vi "Open Port.vi"(7 "timeout":u32=1000, 8 "error in":errorcluster, 9 "Message Cfg":T1={"EnTermChar"=TRUE, "termChar"=10, "suppEnEnRd"=FALSE, "sendEndEn"=FALSE} {"termChar" format="%.0x"}, 10 "serialCfg":T2={"baud rate (9600)"=9600, "data bits (8)"=8, "stop bits (10: 1 bit)"=10, "parity (0:none)"=enum."None", "flow control (0:none)"=0, "endModeforReads"=enum."None", "endModeforWrites"=enum."None"} {"flow control (0:none)" items=["None", "XON/XOFF", "RTS/CTS", "XON/XOFF & RTS/CTS", "DTR/DSR", "XON/XOFF & DTR/DSR"]; "stop bits (10: 1 bit)" items=["1.0"=10, "1.5"=15, "2.0"=20]; "data bits (8)" min=5 max=8 step=1}, 11 "Serial IO in":refnum<class "Serial IO.lvclass">) -> (0 "error out":errorcluster, 3 "Serial IO out":refnum<class "Serial IO.lvclass">)   [LabVIEW 2015, in "Serial IO.lvclass"]
doc: "Open a serial port for communication with a device."
uses:
  Serial IO.lvclass
  Serial IO.lvclass/Serial IO.ctl
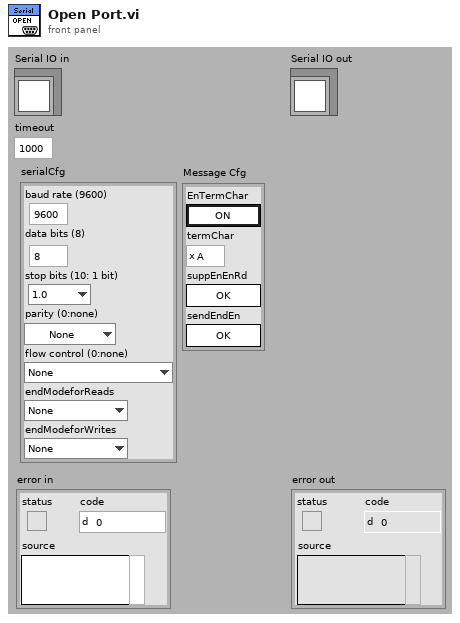
[diagram p1: front panel]
types:
  T1 = cluster{"EnTermChar":bool, "termChar":u8, "suppEnEnRd":bool, "sendEndEn":bool}
  T2 = cluster{"baud rate (9600)":u32, "data bits (8)":u16, "stop bits (10: 1 bit)":u16, "parity (0:none)":enum16{"None", "Odd", "Even", "Mark", "Space"}, "flow control (0:none)":u16, "endModeforReads":enum16{"None", "Last Bit", "TermChar"}, "endModeforWrites":enum16{"None", "Last Bit", "TermChar", "Break"}}
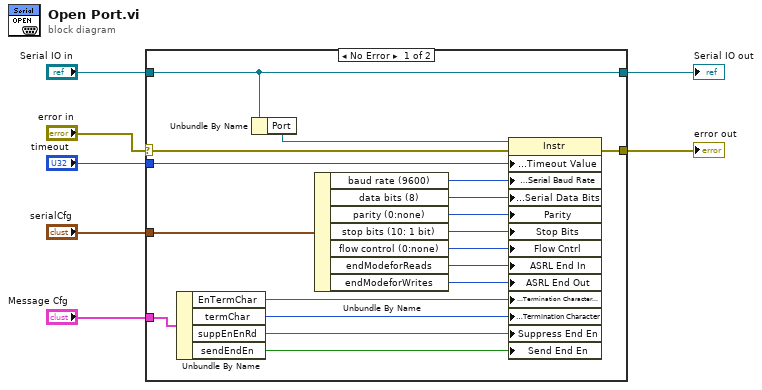
[diagram p0: block diagram]
diagram:
  n1 = case shown="No Error" "error in" {
    selector: "error in" -> [w17 w27]
    tunnel: [w16 w27] -> w6
    tunnel: [w25 w26] -> w4
    tunnel: "Serial IO in" -> [w25 w26]
    tunnel: "serialCfg" -> [w24 _]
    tunnel: "timeout" -> [w15 _]
    tunnel: "Message Cfg" -> [w12 _]
    frame No Error {
      n2 = Unbundle By Name(w12) -> ("EnTermChar"=w11:bool, "termChar"=w10:u8, "suppEnEnRd"=w9:bool, "sendEndEn"=w8:bool)
      n3 = Unbundle By Name(w25) -> ("Port"=w18:refnum<visa-resource-name>)
      n4 = Unbundle By Name(w24) -> ("baud rate (9600)"=w23:u32, "data bits (8)"=w22:u16, "parity (0:none)"=w21:enum16{"None", "Odd", "Even", "Mark", "Space"}, "stop bits (10: 1 bit)"=w20:u16, "flow control (0:none)"=w19:u16, "endModeforReads"=w14:enum16{"None", "Last Bit", "TermChar"}, "endModeforWrites"=w13:enum16{"None", "Last Bit", "TermChar", "Break"})
      n5 = property class="Instr"(reference=w18, error in=w17, "General Settings:Timeout Value"=w15, "Serial Settings:Serial Baud Rate"=w23, "Serial Settings:Serial Data Bits"=w22, "Parity"=w21, "Stop Bits"=w20, "Flow Cntrl"=w19, "ASRL End In"=w14, "ASRL End Out"=w13, "Message Based Settings:Termination Character Enable"=w11, "Message Based Settings:Termination Character"=w10, "Suppress End En"=w9, "Send End En"=w8) -> (error out=w16:errorcluster)  [unwired: 1 in]
    }
    frame Error {
    }
  }
  "error out" <- w6
  "Serial IO out" <- w4
